vi "波形图接受的数据类型.vi"() -> ()   [LabVIEW 2010]
uses:
  Instance           1 27Saved   graph接受的数据类型 .vi
  <vilib>/Analysis/NI_AALBase.lvlib
  <vilib>/measure/NI_MABase.lvlib
panel:
  out "波形图":dynamicdata(graph)
  out "波形图":waveform(dbl)[](graph)
  out "波形图":cluster{i32, i32, cluster{dbl[]}[]}(graph)
  out "波形图":cluster{dbl[]}[](graph)
  out "波形图":cluster{i32, i32, dbl[]}[](graph)
  out "波形图":cluster{i32, i32, dbl[][]}(graph)
  out "波形图":dbl[][](graph)
  out "波形图":cluster{i32, i32, "Sine Wave":dbl[]}(graph)
  out "波形图":dbl[](graph)
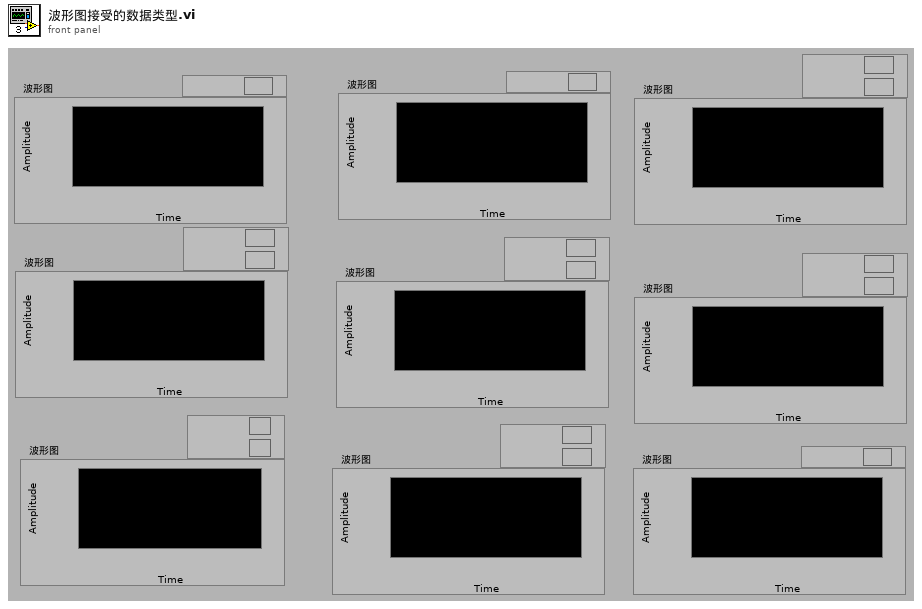
[diagram p1: front panel]
types:
  T1 = cluster{i32, i32, cluster{"square wave":dbl[]}[]}
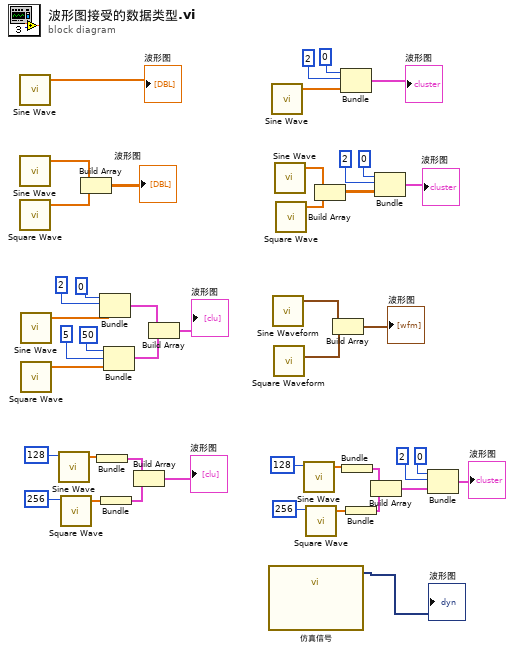
[diagram p0: block diagram]
diagram:
  n1 = call <vilib>:"Sine Wave.vi"() -> ("sine wave"=→"波形图":dbl[])  [unwired: 5 in, 2 out]
  n2 = call <vilib>:"Sine Wave.vi"() -> ("sine wave"=w39:dbl[])  [unwired: 5 in, 2 out]
  n3 = call <vilib>:"Square Wave.vi"() -> ("square wave"=w38:dbl[])  [unwired: 6 in, 2 out]
  n4 = call <vilib>:"Sine Wave.vi"() -> ("sine wave"=w27:dbl[])  [unwired: 5 in, 2 out]
  n5 = call <vilib>:"Square Wave.vi"() -> ("square wave"=w26:dbl[])  [unwired: 6 in, 2 out]
  n6 = call <vilib>:"Sine Wave.vi"("samples"=128) -> ("sine wave"=w18:dbl[])  [unwired: 4 in, 2 out]
  n7 = call <vilib>:"Square Wave.vi"("samples"=256) -> ("square wave"=w19:dbl[])  [unwired: 5 in, 2 out]
  n8 = Build Array(w39, w38) -> (→"波形图":dbl[][])
  n9 = Bundle("sine wave"=w18) -> (w20:cluster{"sine wave":dbl[]})  [unwired: 1 in]
  n10 = Bundle(0, 2, "sine wave"=w27) -> (w24:cluster{i32, i32, "sine wave":dbl[]})  [unwired: 1 in]
  n11 = Bundle("square wave"=w19) -> (w21:cluster{"square wave":dbl[]})  [unwired: 1 in]
  n12 = Bundle(50, 5, "square wave"=w26) -> (w23:cluster{i32, i32, "square wave":dbl[]})  [unwired: 1 in]
  n13 = Build Array(w20, w21) -> (→"波形图":cluster{"square wave":dbl[]}[])
  n14 = Build Array(w24, w23) -> (→"波形图":cluster{i32, i32, "square wave":dbl[]}[])
  n15 = call "仿真信号"() -> ("Signal"=→"波形图":dynamicdata)  [unwired: 14 in, 1 out]
  n16 = call <vilib>:"Sine Wave.vi"() -> ("sine wave"=w41:dbl[])  [unwired: 5 in, 2 out]
  n17 = call <vilib>:"Sine Waveform.vi"() -> ("signal out"=w4:waveform(dbl))  [unwired: 10 in, 1 out]
  n18 = call <vilib>:"Square Waveform.vi"() -> ("signal out"=w3:waveform(dbl))  [unwired: 10 in, 1 out]
  n19 = call <vilib>:"Sine Wave.vi"() -> ("sine wave"=w35:dbl[])  [unwired: 5 in, 2 out]
  n20 = call <vilib>:"Square Wave.vi"() -> ("square wave"=w36:dbl[])  [unwired: 6 in, 2 out]
  n21 = call <vilib>:"Sine Wave.vi"("samples"=128) -> ("sine wave"=w12:dbl[])  [unwired: 4 in, 2 out]
  n22 = call <vilib>:"Square Wave.vi"("samples"=256) -> ("square wave"=w11:dbl[])  [unwired: 5 in, 2 out]
  n23 = Build Array(w35, w36) -> (w32:dbl[][])
  n24 = Build Array(w4, w3) -> (→"波形图":waveform(dbl)[])
  n25 = Bundle(0, 2, "sine wave"=w41) -> (→"波形图":cluster{i32, i32, "sine wave":dbl[]})  [unwired: 1 in]
  n26 = Bundle("sine wave"=w12) -> (w10:cluster{"sine wave":dbl[]})  [unwired: 1 in]
  n27 = Bundle("square wave"=w11) -> (w9:cluster{"square wave":dbl[]})  [unwired: 1 in]
  n28 = Build Array(w10, w9) -> (w8:cluster{"square wave":dbl[]}[])
  n29 = Bundle(0, 2, w32) -> (→"波形图":cluster{i32, i32, dbl[][]})  [unwired: 1 in]
  n30 = Bundle(0, 2, w8) -> (→"波形图":T1)  [unwired: 1 in]
